vi "calc_CurrentpulseWaveform_v0.03.vi"(0 "New input cluster":T1={"Which Position to use for Experiment"=enum."Jumper Safe Position", "Duration (s)"=0.0, "Delay (s)"=0.0, "Pulse 2 (s)"=0.0, "Pulse 1 (pA)"=1.0, "Replicates"=1.0, "Pulse 1 (s)"=1.0, "Pulse 2 (pA)"=0.0, "Iholding (pA)"=0.0, "Valve 1 Position"=2, "Valve 2 Position"=2, "Valve 3 Position"=2, "valve 1 used now?"=TRUE, "valve 2 used now?"=FALSE, "valve 3 used now? "=FALSE, "Maintain Final Voltage until end?"=TRUE, "delta Pulse 1 (pA)"=0.0, "delta Pulse 2 (pA)"=5.0, "Sweeps"=24.0, "Final Pulse 1 (pA)"=0.0, "Final Pulse 2 (pA)"=0.0, "protocol Preview"=[]} {"Final Pulse 2 (pA)" step=0.1; "Final Pulse 1 (pA)" step=0.1; "Sweeps" min=1.0 step=1.0; "delta Pulse 2 (pA)" step=0.1; "Valve 3 Position" min=1 max=8; "Valve 2 Position" min=1 max=8}, 1 "Clear Waveform?":bool, 5 "Old input cluster":T1={"Which Position to use for Experiment"=enum."Jumper Safe Position", "Duration (s)"=0.0, "Delay (s)"=0.0, "Pulse 2 (s)"=0.0, "Pulse 1 (pA)"=1.0, "Replicates"=1.0, "Pulse 1 (s)"=1.0, "Pulse 2 (pA)"=0.0, "Iholding (pA)"=0.0, "Valve 1 Position"=2, "Valve 2 Position"=2, "Valve 3 Position"=2, "valve 1 used now?"=TRUE, "valve 2 used now?"=FALSE, "valve 3 used now? "=FALSE, "Maintain Final Voltage until end?"=TRUE, "delta Pulse 1 (pA)"=0.0, "delta Pulse 2 (pA)"=5.0, "Sweeps"=24.0, "Final Pulse 1 (pA)"=0.0, "Final Pulse 2 (pA)"=0.0, "protocol Preview"=[]} {"Final Pulse 2 (pA)" step=0.1; "Final Pulse 1 (pA)" step=0.1; "Sweeps" min=1.0 step=1.0; "delta Pulse 2 (pA)" step=0.1; "Valve 3 Position" min=1 max=8; "Valve 2 Position" min=1 max=8}, 7 "sample freq":i32=10000, 11 "error in":errorcluster) -> (4 "output cluster":T1={"Which Position to use for Experiment"=enum."Jumper Safe Position", "Duration (s)"=0.0, "Delay (s)"=0.0, "Pulse 2 (s)"=0.0, "Pulse 1 (pA)"=1.0, "Replicates"=1.0, "Pulse 1 (s)"=1.0, "Pulse 2 (pA)"=0.0, "Iholding (pA)"=0.0, "Valve 1 Position"=2, "Valve 2 Position"=2, "Valve 3 Position"=2, "valve 1 used now?"=TRUE, "valve 2 used now?"=FALSE, "valve 3 used now? "=FALSE, "Maintain Final Voltage until end?"=TRUE, "delta Pulse 1 (pA)"=0.0, "delta Pulse 2 (pA)"=5.0, "Sweeps"=24.0, "Final Pulse 1 (pA)"=0.0, "Final Pulse 2 (pA)"=0.0, "protocol Preview"=[]} {"Final Pulse 2 (pA)" step=0.1; "Final Pulse 1 (pA)" step=0.1; "Sweeps" min=1.0 step=1.0; "delta Pulse 2 (pA)" step=0.1; "Valve 3 Position" min=1 max=8; "Valve 2 Position" min=1 max=8}, 15 "error out":errorcluster)   [LabVIEW 2019]
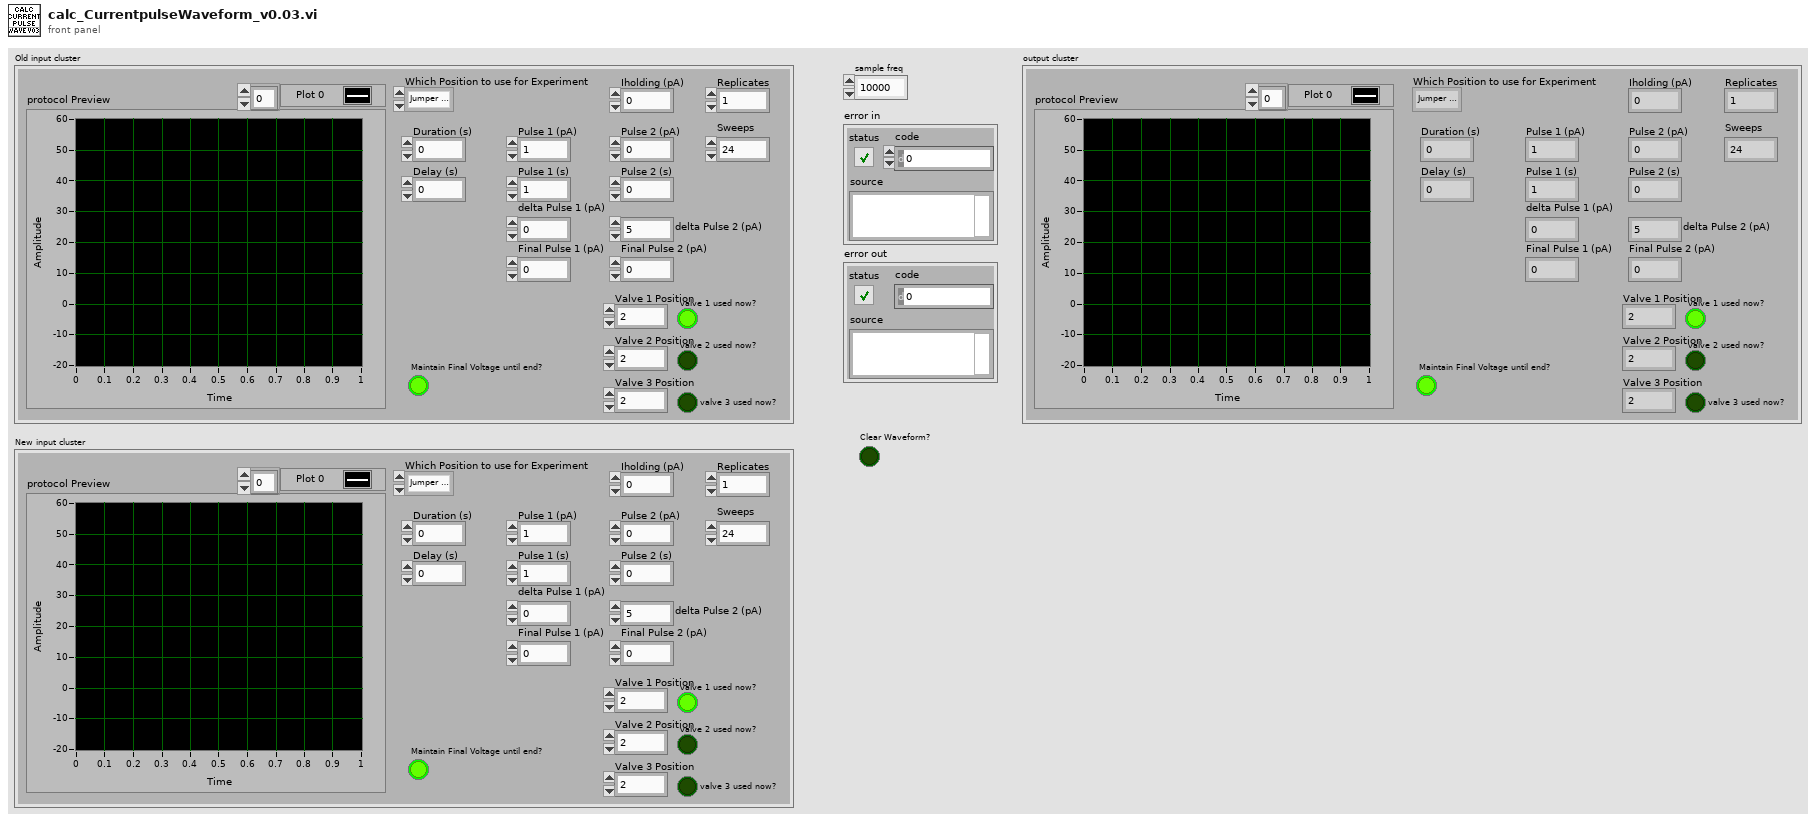
[diagram p1: front panel]
types:
  T1 = cluster{"Which Position to use for Experiment":enum16{"Jumper Safe Position", "Experiment Safe Position", "Jumper Position A", "Jumper Position B", "Jumper Position C", "Jumper Position o-A", "Jumper Position A-o", "Jumper Position A-B", "Jumper Position B-A", "Jumper Position B-C", "Jumper Position C-B", "Jumper Position C-o", "Jumper Position o-C", "Don't Move"}, "Duration (s)":dbl, "Delay (s)":dbl, "Pulse 2 (s)":dbl, "Pulse 1 (pA)":dbl, "Replicates":dbl, "Pulse 1 (s)":dbl, "Pulse 2 (pA)":dbl, "Iholding (pA)":dbl, "Valve 1 Position":i16, "Valve 2 Position":i16, "Valve 3 Position":i16, "valve 1 used now?":bool, "valve 2 used now?":bool, "valve 3 used now? ":bool, "Maintain Final Voltage until end?":bool, "delta Pulse 1 (pA)":dbl, "delta Pulse 2 (pA)":dbl, "Sweeps":dbl, "Final Pulse 1 (pA)":dbl, "Final Pulse 2 (pA)":dbl, "protocol Preview":waveform(dbl)[]}
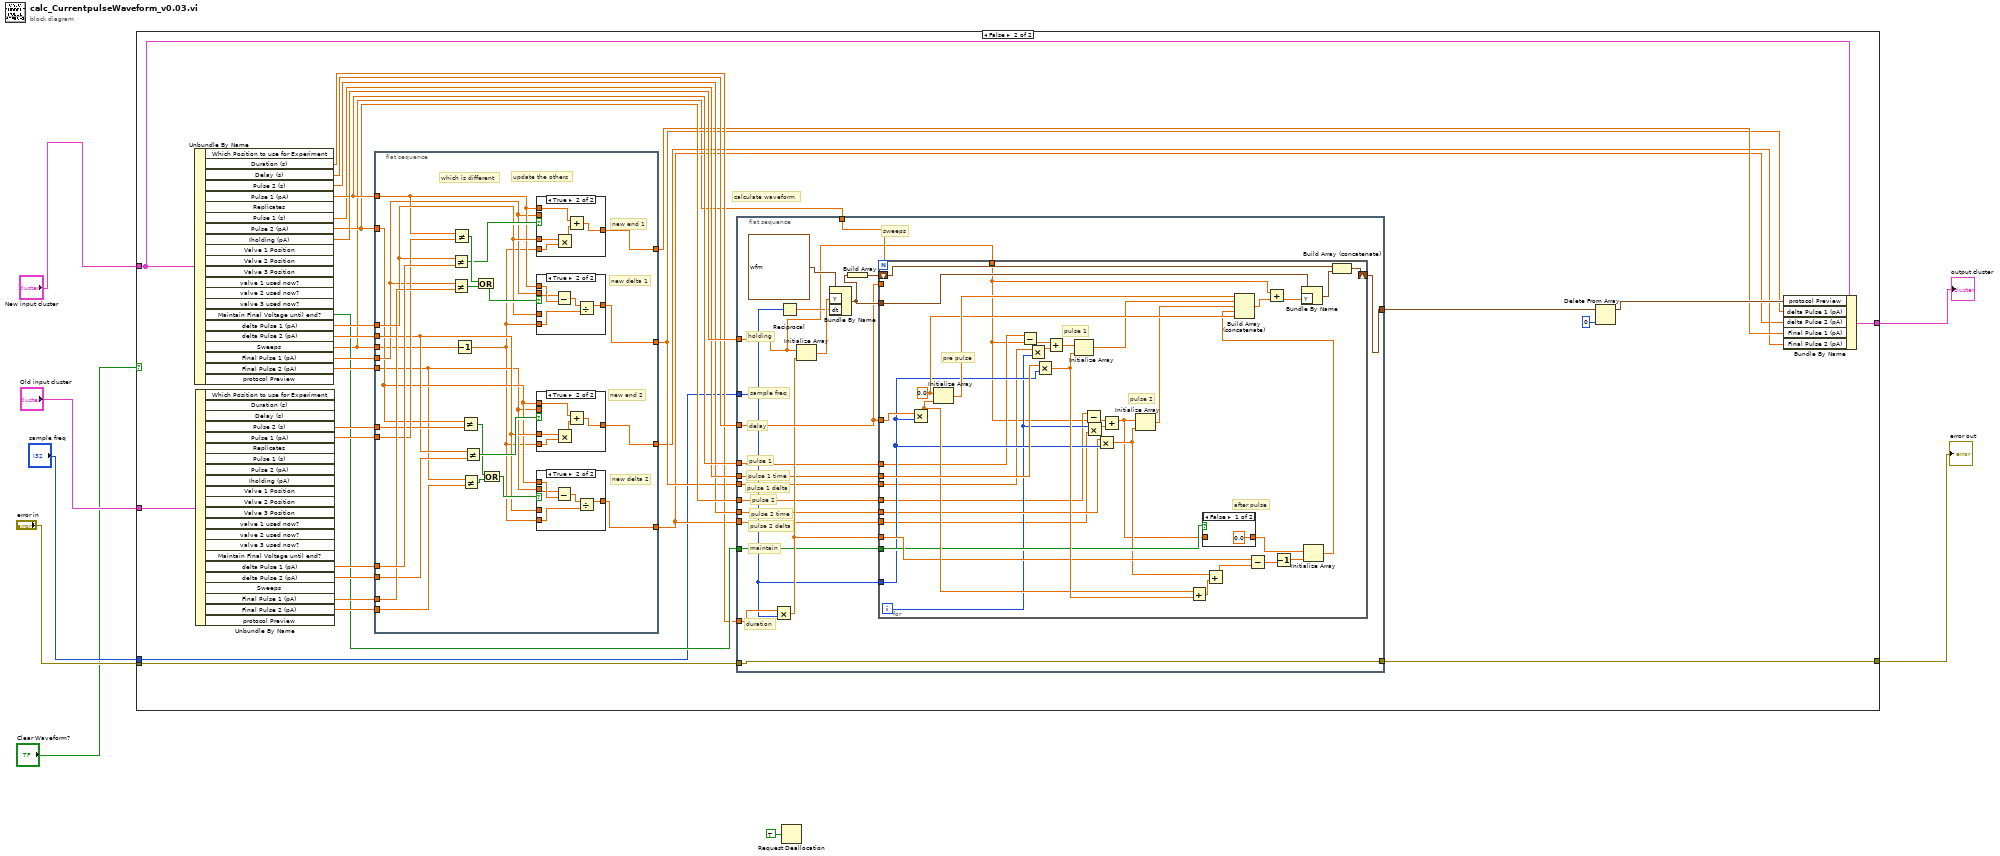
[diagram p0: block diagram]
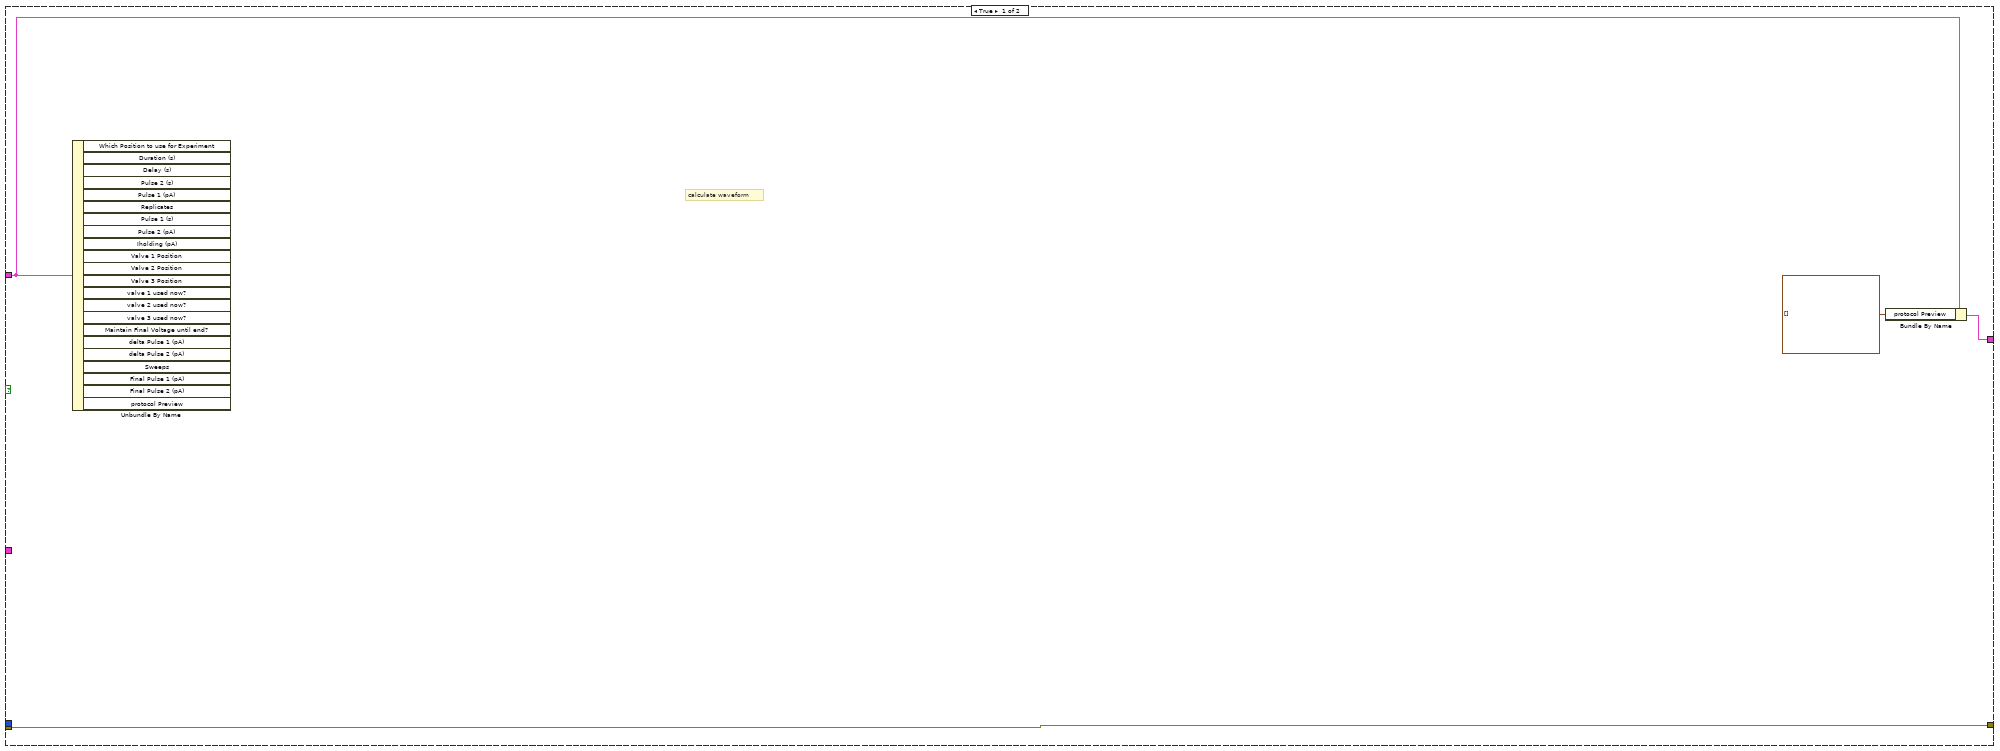
[diagram p2: hidden frame]
diagram:
  n1 = case shown="False" "Clear Waveform?" {
    tunnel: "New input cluster" -> [w12 w44]
    tunnel: [w11 w43] -> w7
    tunnel: "Old input cluster" -> [_ w42]
    tunnel: [w9 w38] -> w5
    tunnel: "error in" -> [w9 w37]
    tunnel: "sample freq" -> [_ w13]
    frame True {
      # "calculate waveform"
      n2 = Unbundle By Name(w12) -> ()  [unwired: 22 out]
      n3 = Bundle By Name(cluster=w12, "protocol Preview"=waveform(dbl)[] []) -> (w11:T1)
    }
    frame False {
      # "calculate waveform"
      n4 = Unbundle By Name(w44) -> ("Duration (s)"=w19:dbl, "Delay (s)"=w27:dbl, "Pulse 2 (s)"=w22:dbl, "Pulse 1 (pA)"=w26:dbl, "Pulse 1 (s)"=w25:dbl, "Pulse 2 (pA)"=w23:dbl, "Iholding (pA)"=w28:dbl, "Maintain Final Voltage until end?"=w20:bool, "delta Pulse 1 (pA)"=w33:dbl, "delta Pulse 2 (pA)"=w29:dbl, "Sweeps"=w14:dbl, "Final Pulse 1 (pA)"=w24:dbl, "Final Pulse 2 (pA)"=w21:dbl)  [unwired: 9 out]
      n5 = Unbundle By Name(w42) -> ("Pulse 2 (s)"=w32:dbl, "Pulse 1 (pA)"=w34:dbl, "delta Pulse 1 (pA)"=w36:dbl, "delta Pulse 2 (pA)"=w31:dbl, "Final Pulse 1 (pA)"=w35:dbl, "Final Pulse 2 (pA)"=w30:dbl)  [unwired: 16 out]
      n6 = flat-sequence {
        tunnel: w36 -> [w70]
        tunnel: w35 -> [w69]
        tunnel: w34 -> [w68]
        tunnel: w33 -> [w63]
        tunnel: w32 -> [w58]
        tunnel: w31 -> [w57]
        tunnel: w30 -> [w46]
        tunnel: w29 -> [w56]
        tunnel: w26 -> [w55]
        tunnel: w24 -> [w54]
        tunnel: w23 -> [w53]
        tunnel: w21 -> [w52]
        tunnel: w14 -> [w51]
        tunnel: [w50] -> w18
        tunnel: [w49] -> w17
        tunnel: [w48] -> w16
        tunnel: [w47] -> w15
        frame #0 {
          # "new delta 2"
          # "new end 2"
          # "new delta 1"
          # "new end 1"
          # "update the others"
          # "which is different"
          n7 = Not Equal?(x=w63, y=w70) -> (x != y?=w64:bool)
          n8 = Not Equal?(x=w54, y=w69) -> (x != y?=w66:bool)
          n9 = Not Equal?(x=w55, y=w68) -> (x != y?=w67:bool)
          n10 = Decrement(x=w51) -> (x-1=w45:dbl)
          n11 = Not Equal?(x=w53, y=w58) -> (x != y?=w59:bool)
          n12 = Not Equal?(x=w52, y=w46) -> (x != y?=w60:bool)
          n13 = Not Equal?(x=w56, y=w57) -> (x != y?=w62:bool)
          n14 = Compound Arithmetic op=OR(w67, w66) -> (w65:bool)
          n15 = Compound Arithmetic op=OR(w59, w60) -> (w61:bool)
          n16 = case shown="True" w64 {
            tunnel: w55 -> [_ w91]
            tunnel: w45 -> [_ w93]
            tunnel: w54 -> [w89 _]
            tunnel: w63 -> [_ w94]
            tunnel: [w89 w90] -> w50
            frame False {
            }
            frame True {
              n17 = Multiply(x=w94, y=w93) -> (x*y=w92:dbl)
              n18 = Add(x=w91, y=w92) -> (x+y=w90:dbl)
            }
          }
          n19 = case shown="True" w65 {
            tunnel: w55 -> [_ w88]
            tunnel: w54 -> [_ w87]
            tunnel: w63 -> [w83 _]
            tunnel: w45 -> [_ w84]
            tunnel: [w83 w85] -> w49
            frame False {
            }
            frame True {
              n20 = Subtract(x=w87, y=w88) -> (x-y=w86:dbl)
              n21 = Divide(x=w86, y=w84) -> (x/y=w85:dbl)
            }
          }
          n22 = case shown="True" w62 {
            tunnel: w53 -> [_ w79]
            tunnel: w45 -> [_ w81]
            tunnel: w52 -> [w77 _]
            tunnel: w56 -> [_ w82]
            tunnel: [w77 w78] -> w48
            frame False {
            }
            frame True {
              n23 = Multiply(x=w82, y=w81) -> (x*y=w80:dbl)
              n24 = Add(x=w79, y=w80) -> (x+y=w78:dbl)
            }
          }
          n25 = case shown="True" w61 {
            tunnel: w53 -> [_ w76]
            tunnel: w52 -> [_ w75]
            tunnel: w56 -> [w71 _]
            tunnel: w45 -> [_ w72]
            tunnel: [w71 w73] -> w47
            frame False {
            }
            frame True {
              n26 = Subtract(x=w75, y=w76) -> (x-y=w74:dbl)
              n27 = Divide(x=w74, y=w72) -> (x/y=w73:dbl)
            }
          }
        }
      }
      n28 = flat-sequence {
        tunnel: w19 -> [w106]
        tunnel: w37 -> [w96]
        tunnel: w27 -> [w109]
        tunnel: w26 -> [w102]
        tunnel: w14 -> [w114]
        tunnel: w13 -> [w95]
        tunnel: w28 -> [w107]
        tunnel: w25 -> [w101]
        tunnel: w23 -> [w100]
        tunnel: w17 -> [w104]
        tunnel: w20 -> [w103]
        tunnel: w22 -> [w99]
        tunnel: w15 -> [w98]
        tunnel: [w97] -> w40
        tunnel: [w96] -> w38
        frame #0 {
          # "duration"
          # "maintain"
          # "pulse 2 delta"
          # "pulse 2 time"
          # "pulse 2"
          # "pulse 1 delta"
          # "pulse 1 time"
          # "pulse 1"
          # "delay"
          # "sample freq"
          # "sweeps"
          # "holding"
          n29 = Multiply(x=w106, y=w95) -> (x*y=w105:dbl)
          n30 = Reciprocal(x=w95) -> (1/x=w108:dbl)
          n31 = Initialize Array(w107, w105) -> (w111:dbl[])
          n32 = Bundle By Name(cluster=waveform(dbl) {"t0"=timestamp(0 s since 1904-01-01), "dt"=1.0, "Y"=[]} ("signal out"), "Y"=w111, "dt"=w108) -> (w110:waveform(dbl))
          n33 = Build Array(w110) -> (w113:waveform(dbl)[])
          n34 = for {
            N: w114 -> [_]
            tunnel: w109 -> [_]
            shift-right: [w151] -> w97
            shift-left: w113 -> [w150]
            tunnel: w110 -> [w148]
            tunnel: w102 -> [w119]
            tunnel: w109 -> [w145]
            tunnel: w101 -> [w144]
            tunnel: w107 -> [w115]
            tunnel: w95 -> [w132]
            tunnel: w104 -> [w125]
            tunnel: w105 -> [w138]
            tunnel: w103 -> [w134]
            tunnel: w100 -> [w117]
            tunnel: w99 -> [w131]
            tunnel: w98 -> [w121]
            i -> [w123]
            w143 = 0.0 ("element")
            # "after pulse"
            # "pulse 2"
            # "pulse 1"
            # "pre pulse"
            n35 = Multiply(x=w145, y=w132) -> (x*y=w139:dbl)
            n36 = Initialize Array(w143, w139) -> (w147:dbl[])
            n37 = Subtract(x=w119, y=w115) -> (x-y=w120:dbl)
            n38 = Multiply(x=w125, y=w123) -> (x*y=w126:dbl)
            n39 = Multiply(x=w144, y=w132) -> (x*y=w140:dbl)
            n40 = Add(x=w120, y=w126) -> (x+y=w127:dbl)
            n41 = Initialize Array(w127, w140) -> (w133:dbl[])
            n42 = Subtract(x=w117, y=w115) -> (x-y=w118:dbl)
            n43 = Multiply(x=w123, y=w121) -> (x*y=w122:dbl)
            n44 = Multiply(x=w131, y=w132) -> (x*y=w129:dbl)
            n45 = Add(x=w118, y=w122) -> (x+y=w124:dbl)
            n46 = Initialize Array(w124, w129) -> (w128:dbl[])
            n47 = Add(x=w139, y=w140) -> (x+y=w146:dbl)
            n48 = case shown="False" w134 {
              tunnel: w124 -> [_ w153]
              tunnel: [0.0 w153] -> w135
              frame False {
              }
              frame True {
              }
            }
            n49 = Add(x=w129, y=w146) -> (x+y=w130:dbl)
            n50 = Subtract(x=w138, y=w130) -> (x-y=w137:dbl)
            n51 = Decrement(x=w137) -> (x-1=w141:dbl)
            n52 = Initialize Array(w135, w141) -> (w142:dbl[])
            n53 = Build Array (concatenate)(w147, w133, w128, w142, w143) -> (w136:dbl[])
            n54 = Add(x=w115, y=w136) -> (x+y=w116:dbl[])
            n55 = Bundle By Name(cluster=w148, "Y"=w116) -> (w149:waveform(dbl))
            n56 = Build Array (concatenate)(w150, w149) -> (w151:waveform(dbl)[])
          }
        }
      }
      n57 = Delete From Array(array=w40, index=0) -> (array with subset deleted=w39:waveform(dbl)[])  [unwired: 1 in, 1 out]
      n58 = Bundle By Name(cluster=w44, "protocol Preview"=w39, "delta Pulse 1 (pA)"=w17, "delta Pulse 2 (pA)"=w15, "Final Pulse 1 (pA)"=w18, "Final Pulse 2 (pA)"=w16) -> (w43:T1)
    }
  }
  "output cluster" <- w7
  "error out" <- w5
  n59 = Request Deallocation(TRUE ("flag")) -> ()
